vi "Fetch - Variant.vi"(7 "PV name":string, 8 "error in":errorcluster, 10 "default value":variant, 11 "Server in":refnum<class "Server.lvclass">) -> (0 "error out":errorcluster, 1 "PV not found?":bool, 2 "value":variant, 3 "Server out":refnum<class "Server.lvclass">)   [LabVIEW 2020, in "PV Access.lvlib" / "PVA Server.lvlib" / "Server.lvclass"]
uses:
  Server.lvclass
  Server.lvclass/Server.ctl
  Source/Source.lvclass
  PV Data/PV Data/PV Data.lvclass
  PV Data/PV Data/Read Field - Variant.vi
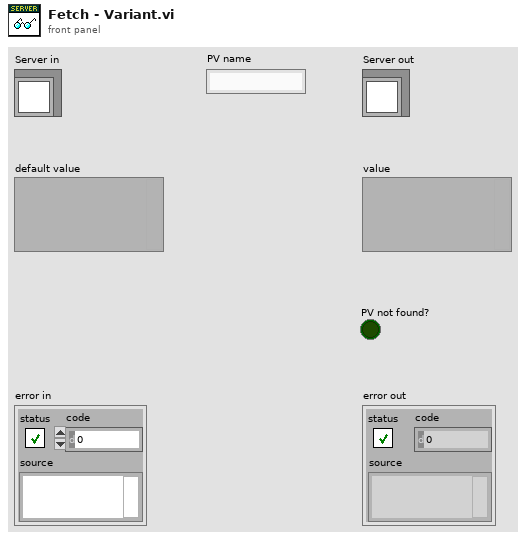
[diagram p1: front panel]
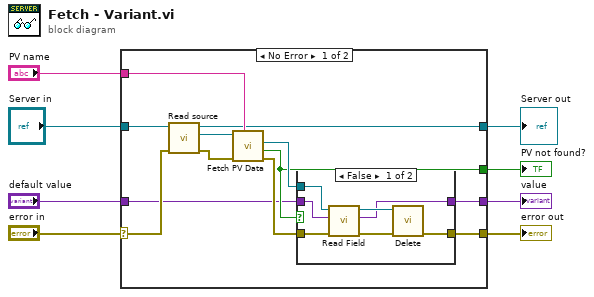
[diagram p0: block diagram]
diagram:
  n1 = case shown="No Error" "error in" {
    selector: "error in" -> [w19 w30]
    tunnel: [w9 w30] -> w8
    tunnel: "PV name" -> [w20 _]
    tunnel: "Server in" -> [w17 w32]
    tunnel: [w16 w32] -> w4
    tunnel: "default value" -> [w11 w31]
    tunnel: [w10 w31] -> w2
    tunnel: [w12 _] -> w1
    frame No Error {
      n2 = call "Read source.vi"("error in (no error)"=w19, "Server in"=w17) -> ("error out"=w18:errorcluster, "Source"=w15:refnum<class "Source.lvclass">, "Server out"=w16:refnum<class "Server.lvclass">)  [unwired: 7 in]
      n3 = call "Fetch PV Data.vi"("PV name"=w20, "error in"=w18, "Source in"=w15) -> ("error out"=w14:errorcluster, "PV not found?"=w12:bool, "PV Data out"=w13:refnum<class "PV Data.lvclass">)  [unwired: 5 in, 1 out]
      n4 = case shown="False" w12 {
        tunnel: w14 -> [w27 w28]
        tunnel: w13 -> [w25 _]
        tunnel: w11 -> [w23 w29]
        tunnel: [w22 w29] -> w10
        tunnel: [w21 w28] -> w9
        frame False {
          n5 = call-poly "Read Field.vi"("error in (no error)"=w27, "value"=w23, "PV Data in"=w25) -> ("error out"=w26:errorcluster, "value out"=w22:variant, "PV Data out"=w24:refnum<class "PV Data.lvclass">)  [unwired: 5 in, 1 out]
          n6 = call "Delete.vi"("error in (no error)"=w26, "PV Data in"=w24) -> ("error out"=w21:errorcluster)  [unwired: 9 in]
        }
        frame True {
        }
      }
    }
    frame Error {
    }
  }
  "Server out" <- w4
  "error out" <- w8
  "value" <- w2
  "PV not found?" <- w1
